vi "Read Device Name.vi"(8 "error in (no error)":errorcluster, 11 "Analog in":refnum<class "Hardware.lvclass">) -> (0 "error out":errorcluster, 2 "Device Name":string, 3 "Analog out":refnum<class "Hardware.lvclass">)   [LabVIEW 2019, in "Hardware.lvlib" / "Hardware.lvclass"]
uses:
  Hardware.lvclass
  Hardware.lvclass/Hardware.ctl
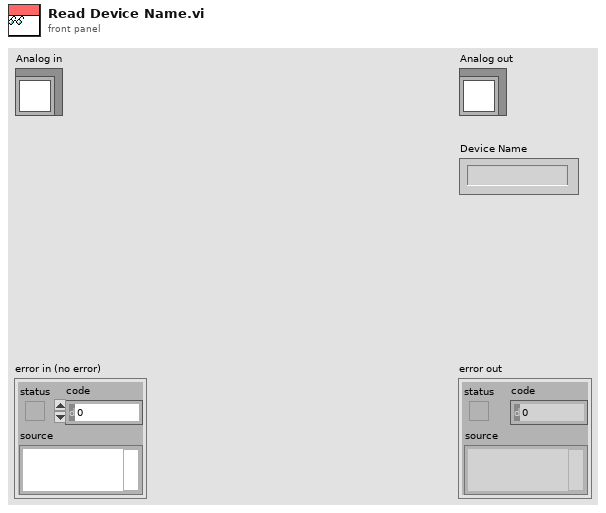
[diagram p1: front panel]
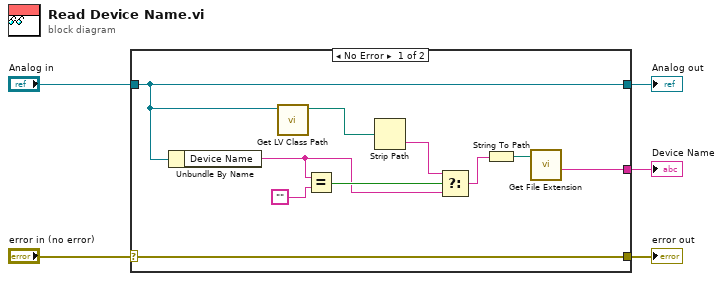
[diagram p0: block diagram]
diagram:
  n1 = case shown="No Error" "error in (no error)" {
    selector: "error in (no error)" -> [w15 w16]
    tunnel: [w15 w16] -> w4
    tunnel: [w9 w17] -> w2
    tunnel: "Analog in" -> [w9 w17]
    tunnel: [w6 _] -> w1
    frame No Error {
      n2 = Unbundle By Name(w9) -> ("Device Name"=w12:string)
      n3 = call <vilib>:"Get LV Class Path.vi"("object"=w9) -> ("class path"=w10:path)  [unwired: 9 in, 1 out]
      n4 = Equal?(x=w12, y="") -> (x = y?=w13:bool)
      n5 = Strip Path(path=w10) -> (name=w11:string)  [unwired: 1 out]
      n6 = Select(t=w11, s=w13, f=w12) -> (s? t:f=w7:string)
      n7 = String To Path(string=w7) -> (path=w8:path)
      n8 = call <vilib>:"Get File Extension.vi"("file"=w8) -> ("filename without extension"=w6:string)  [unwired: 6 in, 4 out]
    }
    frame Error {
    }
  }
  "error out" <- w4
  "Analog out" <- w2
  "Device Name" <- w1
